vi "Deterministic Errors.Set Error Description.vi"(10 "error description":string, 11 "error in":errorcluster) -> (1 "new offset":i32, 3 "error out":errorcluster)   [LabVIEW 2016, in "Deterministic Errors.lvlib"]
uses:
  Deterministic Errors.lvlib
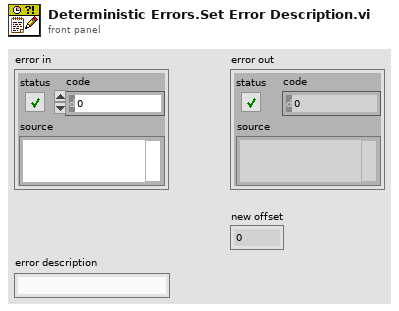
[diagram p1: front panel]
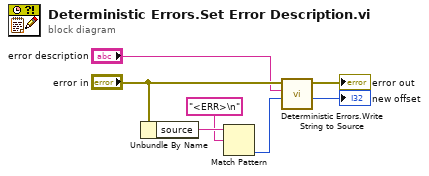
[diagram p0: block diagram]
diagram:
  n1 = Unbundle By Name("error in") -> ("source"=w7:string)
  n2 = Match Pattern(string=w7, regular expression="<ERR>\n") -> (offset past match=w2:i32)  [unwired: 1 in, 3 out]
  n3 = call "Deterministic Errors.Write String to Source.vi"("offset (0)"=w2, "string"="error description", "error in"="error in") -> ("new offset"=→"new offset":i32, "error out"=→"error out":errorcluster)  [unwired: 7 in]
